vi "Status Position.vi"(8 "error in (no error)":errorcluster, 11 "status":i32) -> (0 "error out":errorcluster, 2 "function return":i32, 3 "status out":i32)   [LabVIEW 2020, in "ThorECU.lvlib"]
doc: "long StatusPosition(long &status);"
uses:
  ThorECU.lvlib
  ThorECU.dll
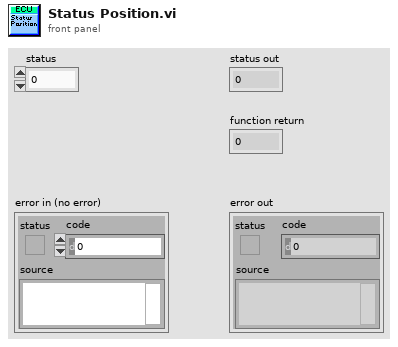
[diagram p1: front panel]
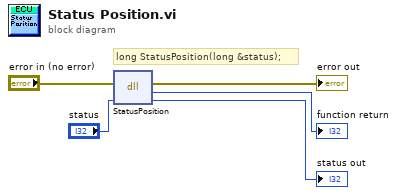
[diagram p0: block diagram]
diagram:
  # "long StatusPosition(long &status);"
  n1 = dll-call lib="D:/software/TweezerTron Project/Instruments/Thorlabs/ECU_SDK/ThorECU.*" fn="StatusPosition"(error in="error in (no error)", "status"="status") -> (error out=→"error out":errorcluster, →"function return":i32, "status"=→"status out":i32)  [unwired: 2 in, 1 out]
